vi "Rad -Deg.vi"(1 "Radians iN":dbl) -> (0 "Degrees out":dbl)   [LabVIEW 2019, in "Exaprom PDF.lvlib"]
uses:
  Exaprom PDF.lvlib
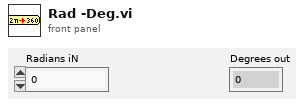
[diagram p1: front panel]
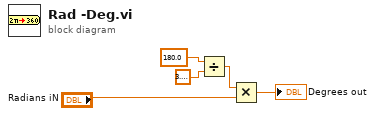
[diagram p0: block diagram]
diagram:
  n1 = Divide(x=180.0 ("y"), y=3.141592653589793) -> (x/y=w5:dbl)
  n2 = Multiply(x=w5, y="Radians iN") -> (x*y=→"Degrees out":dbl)
